vi "Write Optional Plane Labels Visible.vi"(8 "error in (no error)":errorcluster, 10 "OptionalLabelsVisible":bool, 11 "XYGraph.lvclass in":refnum<class "XYGraph.lvclass">) -> (0 "error out":errorcluster, 3 "XYGraph.lvclass out":refnum<class "XYGraph.lvclass">)   [LabVIEW 2015, in "XYGraph.lvclass"]
uses:
  XYGraph.lvclass
  XYGraph.lvclass/XYGraph.ctl
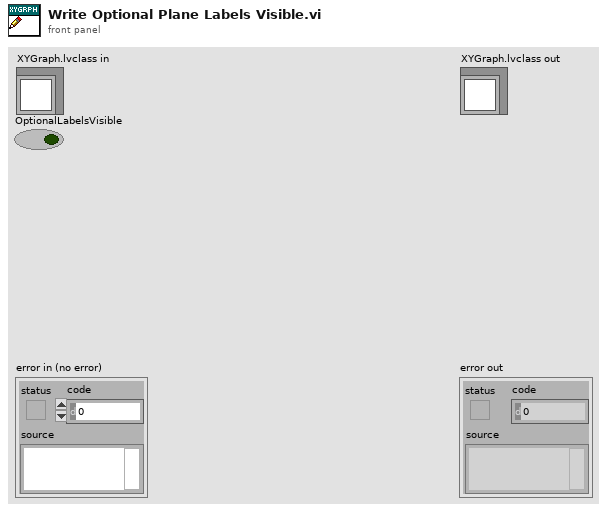
[diagram p1: front panel]
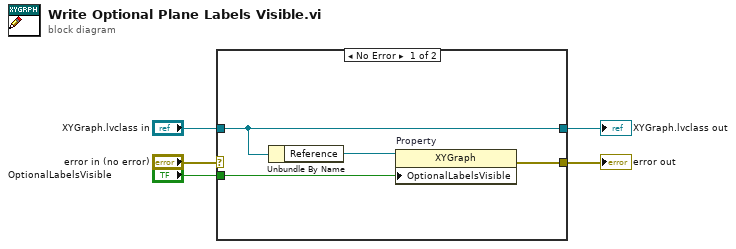
[diagram p0: block diagram]
diagram:
  n1 = case shown="No Error" "error in (no error)" {
    selector: "error in (no error)" -> [_ w11]
    tunnel: [w9 w11] -> w4
    tunnel: [w7 w10] -> w2
    tunnel: "XYGraph.lvclass in" -> [w7 w10]
    tunnel: "OptionalLabelsVisible" -> [w8 _]
    frame No Error {
      n2 = Unbundle By Name(w7) -> ("Reference"=w6:refnum<vi>)
      n3 = property on="Property" class="XYGraph"(reference=w6, "OptionalLabelsVisible"=w8) -> (error out=w9:errorcluster)  [unwired: 1 in, 1 out]
    }
    frame Error {
    }
  }
  "error out" <- w4
  "XYGraph.lvclass out" <- w2
